vi "Alp Led Inquire.vi"(7 "UserVarPtr":i32, 8 "error in (no error)":errorcluster, 9 "InquireType":i32, 10 "LedId":u32, 11 "DeviceId":u32) -> (0 "error out":errorcluster, 3 "function return":i32, 5 "UserVarPtr out":i32)   [LabVIEW 2013, in "alpD41.lvlib"]
doc: "ALP_API long ALP_ATTR AlpLedInquire( ALP_ID DeviceId, ALP_ID LedId, long InquireType, long *UserVarPtr );"
uses:
  <userlib>/alpD41/alpD41.lvlib
  <userlib>/alpD41/alpD41.dll
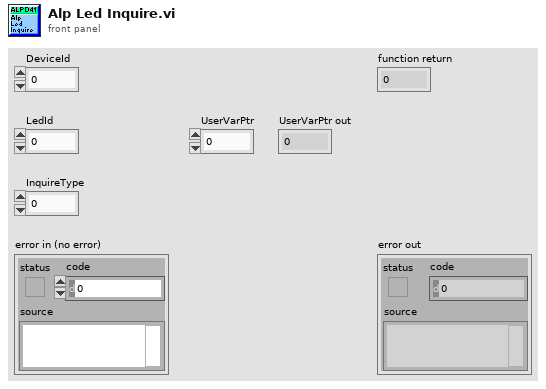
[diagram p1: front panel]
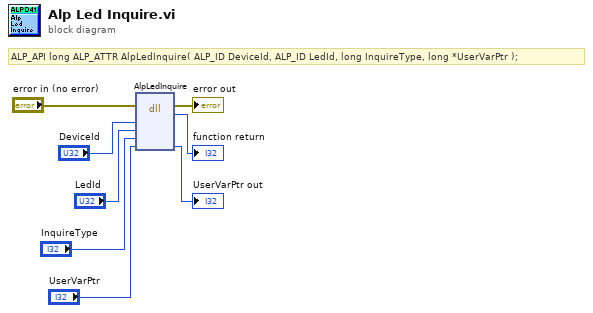
[diagram p0: block diagram]
diagram:
  # "ALP_API long ALP_ATTR AlpLedInquire( ALP_ID DeviceId, ALP_ID LedId, long InquireType, long *UserVarPtr );"
  n1 = dll-call lib="C:/Program Files (x86)/National Instruments/LabVIEW 2013/user.lib/alpD41/alpD41.*" fn="AlpLedInquire"(error in="error in (no error)", "DeviceId"="DeviceId", "LedId"="LedId", "InquireType"="InquireType", "UserVarPtr"="UserVarPtr") -> (error out=→"error out":errorcluster, →"function return":i32, "UserVarPtr"=→"UserVarPtr out":i32)  [unwired: 5 in, 1 out]
